vi "Configure Hardware.vi"(8 "error in (no error)":cluster{"状态":bool, "代码":i32, "源":string} caption="错误输入（无错误）", 11 "硬件资源输入":T1) -> (0 "error out":cluster{"状态":bool, "代码":i32, "源":string} caption="错误输出", 3 "硬件资源输出":T1)   [LabVIEW 2014, in "Acquisition.lvlib"]
doc: "配置硬件。"
uses:
  Acquisition.lvlib
  Hardware Configuration.ctl
  Signal Type.ctl
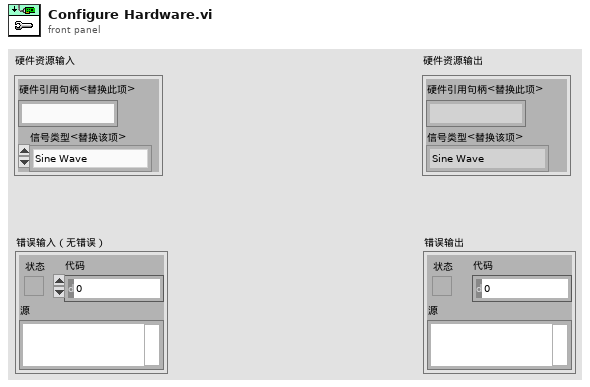
[diagram p1: front panel]
types:
  T1 = typedef "Acquisition.lvlib/Hardware Configuration.ctl" = cluster{"硬件引用句柄<替换此项>":string, "信号类型<替换该项>":T2}
  T2 = typedef "Acquisition.lvlib/Signal Type.ctl" = enum16{"Sine Wave", "Square with Noise"}
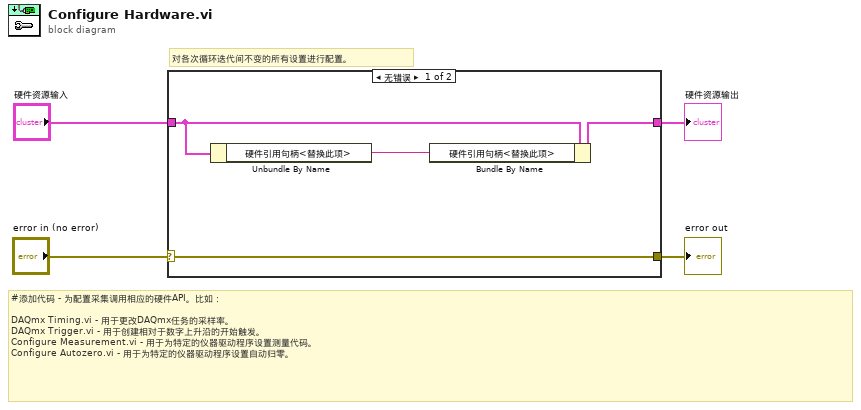
[diagram p0: block diagram]
diagram:
  # "对各次循环迭代间不变的所有设置进行配置。"
  # "#添加代码 - 为配置采集调用相应的硬件API。比如：\n\nDAQmx Timing.vi - 用于更改DAQmx任务的采样率。\nDAQmx Trigger.vi - 用于创建相对于数字上升沿的开始触发。\nConfigure Measurement.vi - 用于为特定的仪器驱动程序设置测量代码。\nConfigure Autozero.vi - 用于为特定的仪器驱动程序设置自动归零。"
  n1 = case shown="无错误" "error in (no error)" {
    selector: "error in (no error)" -> [w7 w9]
    tunnel: [w7 w9] -> w3
    tunnel: "硬件资源输入" -> [w6 w10]
    tunnel: [w8 w10] -> w1
    frame No Error {
      n2 = Unbundle By Name(w6) -> ("硬件引用句柄<替换此项>"=w5:string)
      n3 = Bundle By Name(cluster=w6, "硬件引用句柄<替换此项>"=w5) -> (w8:T1)
    }
    frame Error {
    }
  }
  "硬件资源输出" <- w1
  "error out" <- w3
